vi "CONV 1D Boolean Array to String.vi"(0 "1-D Boolean":bool[](array[boolean]), 1 "Delimiter (,)":string=",", 5 "Boolean Type (1,0)":T1) -> (6 "String":string)   [LabVIEW 2012]
doc: "This routine converts a 1-D Boolean Array into a string list. Boolean False is \"0\", Boolean True is \"1\". The delimiter may be one or more characters."
uses:
  Type Defs/CONV Boolean Type Enum.ctl
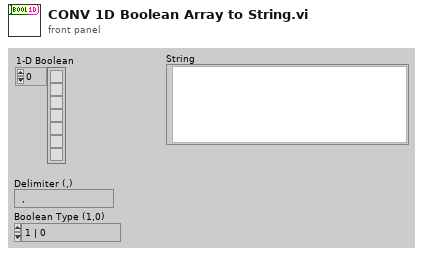
[diagram p1: front panel]
types:
  T1 = typedef "CONV Boolean Type Enum.ctl" = enum16{"1 | 0", "T | F", "True | False", "On | Off", "Yes | No"}
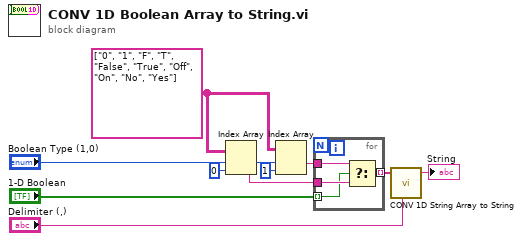
[diagram p0: block diagram]
diagram:
  w7 = string[][] [["0", "1"], ["F", "T"], ["False", "True"], ["Off", "On"], ["No", "Yes"]]
  n1 = Index Array(array=w7, index (row)="Boolean Type (1,0)", index (col)=0) -> (element=w3:string)
  n2 = Index Array(array=w7, index (row)="Boolean Type (1,0)", index (col)=1) -> (element=w2:string)
  n3 = for {
    tunnel: "1-D Boolean" -> [w12] mode=indexing
    tunnel: w3 -> [w13]
    tunnel: w2 -> [w14]
    tunnel: [w11] -> w1 mode=indexing
    n4 = Select(t=w14, s=w12, f=w13) -> (s? t:f=w11:string)
  }
  n5 = call "CONV 1D String Array to String.vi"("1-D String"=w1, "Delimiter (,)"="Delimiter (,)") -> ("String"=→"String":string)  [unwired: 7 out]
